vi "DB_Connect.vi"() -> ()   [LabVIEW 2020]
uses:
  <vilib>/addons/database/Connection.llb/DB Tools Open Connec (String).vi
  <vilib>/addons/database/NI_Database_API.lvlib
panel:
  out "error out":errorcluster
  out "tables":string[](array[string])
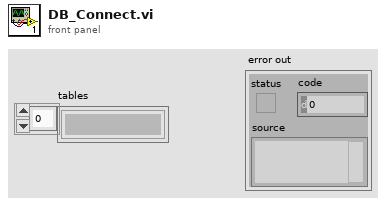
[diagram p1: front panel]
types:
  T1 = typedef "NI_Database_API.lvlib/Conn ObjectReference.ctl" = refnum<k1>
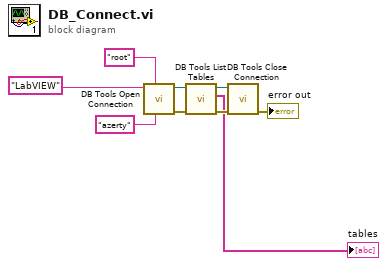
[diagram p0: block diagram]
diagram:
  n1 = call-poly <vilib>:"DB Tools Open Connection.vi"("password"="azerty", "userID"="root", "connection information"="LabVIEW") -> ("error out"=w8:errorcluster, "connection reference"=w9:T1)  [unwired: 5 in]
  n2 = call <vilib>:"DB Tools List Tables.vi"("error in (no error)"=w8, "connection reference"=w9) -> ("error out"=w6:errorcluster, "tables"=→"tables":string[], "connection reference out"=w7:T1)  [unwired: 3 in]
  n3 = call <vilib>:"DB Tools Close Connection.vi"("error in (no error)"=w6, "connection reference"=w7) -> ("error out"=→"error out":errorcluster)  [unwired: 5 in]
